vi "Configure Transmit Parameters.vi"(7 "Micropulse # In":i32, 8 "error in (no error)":errorcluster, 9 "Transmit Parameters":T1 {"Pulse Shape"."Width" min=16 max=1010 step=50 format="%.0fns"}, 10 "Tx Channel":u32) -> (0 "error out":errorcluster, 5 "Micropulse # Out":i32)   [LabVIEW 2026, in "MicroPulse_Driver.lvlib"]
uses:
  MicroPulse_Driver.lvlib
  <instrlib>/MicroPulse/Public/Data/Datatypes/MP - transmit parameters.ctl
  <instrlib>/MicroPulse/Public/Data/Datatypes/MP - pulser voltage.ctl
  <instrlib>/MicroPulse/Public/Data/Datatypes/MP - pulse damping.ctl
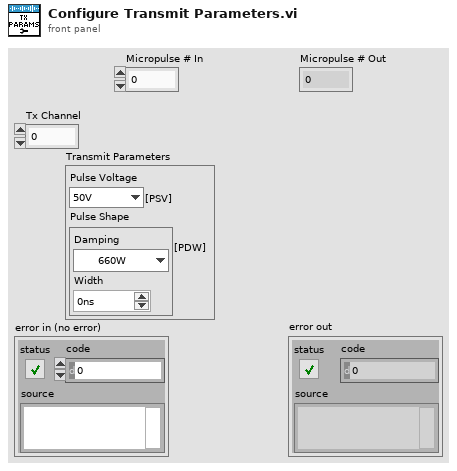
[diagram p1: front panel]
types:
  T1 = typedef "MicroPulse_Driver.lvlib/MP - transmit parameters.ctl" = cluster{"Pulse Voltage":T2, "Pulse Shape":cluster{"Damping":T3, "Width":u32}}
  T2 = typedef "MicroPulse_Driver.lvlib/MP - pulser voltage.ctl" = enum16{"50V", "100V", "150V", "200V", "250V", "300V"}
  T3 = typedef "MicroPulse_Driver.lvlib/MP - pulse damping.ctl" = enum16{"660W", "458W", "220W", "149W", "102W", "82W", "63W", "51W"}
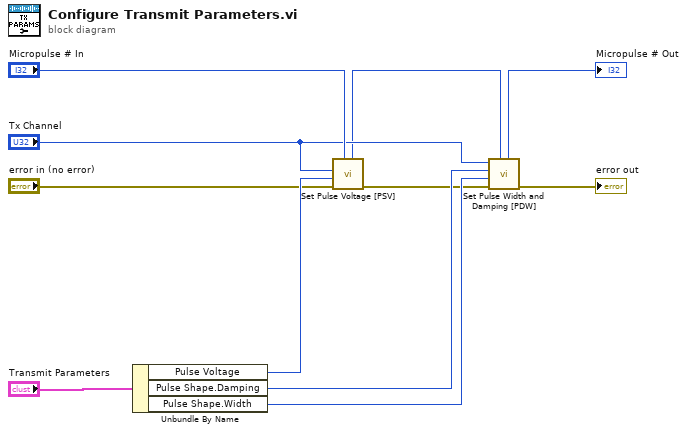
[diagram p0: block diagram]
diagram:
  n1 = Unbundle By Name("Transmit Parameters") -> ("Pulse Voltage"=w6:T2, "Pulse Shape.Damping"=w8:T3, "Pulse Shape.Width"=w9:u32)
  n2 = call "Set Pulse Voltage [PSV].vi"("Micropulse # In"="Micropulse # In", "error in (no error)"="error in (no error)", "Voltage"=w6, "Channel Number"="Tx Channel") -> ("error out"=w1:errorcluster, "Micropulse # Out"=w2:i32)  [unwired: 6 in]
  n3 = call "Set Pulse Width and Damping [PDW].vi"("Micropulse # In"=w2, "error in (no error)"=w1, "Width (ns)"=w9, "Damping"=w8, "Channel Number"="Tx Channel") -> ("error out"=→"error out":errorcluster, "Micropulse # Out"=→"Micropulse # Out":i32)  [unwired: 5 in]
